vi "Interpolate V-I curve.vi"(3 "Input axes. True: V vs I; False: I vs V":bool=TRUE, 4 "Number of V-sweep periods":dbl=1.0, 5 "Index of desired plot":i32, 6 "Input Multiplot":cluster{dbl[], dbl[]}[](graph)=[{array[601 elements], array[601 elements]}, {[-7e-09, -6.976666666666667e-09, -6.953333333333333e-09, -6.93e-09, -6.906666666666667e-09, -6.883333333333333e-09, -6.86e-09, -6.836666666666667e-09, -6.813333333333333e-09, -6.79e-09, -6.766666666666666e-09, -6.743333333333333e-09, -6.72e-09, -6.696666666666666e-09, -6.673333333333333e-09, -6.65e-09, -6.626666666666666e-09, -6.603333333333333e-09, -6.58e-09, -6.556666666666666e-09, -6.533333333333333e-09, -6.51e-09, -6.486666666666666e-09, -6.463333333333333e-09, -6.44e-09, -6.416666666666666e-09, -6.393333333333333e-09, -6.37e-09, -6.346666666666666e-09, -6.323333333333333e-09, -6.3e-09, -6.276666666666666e-09, -6.253333333333333e-09, -6.23e-09, -6.206666666666666e-09, -6.183333333333333e-09, -6.16e-09, -6.136666666666666e-09, -6.113333333333333e-09, -6.09e-09, -6.066666666666666e-09, -6.043333333333333e-09, -6.02e-09, -5.9966666666666664e-09, -5.973333333333333e-09, -5.9499999999999995e-09, -5.9266666666666665e-09, -5.9033333333333334e-09, -5.8799999999999995e-09, -5.8566666666666665e-09, -5.833333333333333e-09, -5.8099999999999996e-09, -5.7866666666666665e-09, -5.763333333333333e-09, -5.74e-09, -5.7166666666666666e-09, -5.693333333333333e-09, -5.67e-09, -5.646666666666667e-09, -5.623333333333333e-09, -5.6e-09, -5.576666666666667e-09, -5.553333333333333e-09, -5.53e-09, -5.506666666666667e-09, -5.483333333333333e-09, -5.46e-09, -5.436666666666667e-09, -5.413333333333333e-09, -5.39e-09, -5.366666666666667e-09, -5.343333333333333e-09, -5.32e-09, -5.296666666666667e-09, -5.273333333333333e-09], [-0.0004821561460872206, -0.00047938288334669894, -0.0004789074718402786, -0.0004777379416474081, -0.000475052203857136, -0.00047223609393540406, -0.00047195794806430995, -0.0004706001620611257, -0.00046771079567058956, -0.0004666969301809305, -0.00046440072995060437, -0.00046159074960749647, -0.0004603654022456595, -0.00045960525980296877, -0.0004591186437168279, -0.00045718015199764495, -0.00045405957870414866, -0.00045358976275954613, -0.00045141277699479917, -0.00044926701129684773, -0.00044740158603609226, -0.00044689019117776554, -0.00044619043907049053, -0.0004433306418334057, -0.00044036373125306503, -0.0004390323537054179, -0.0004379883109219583, -0.0004348498737591965, -0.0004331149798360703, -0.0004325833412496541, -0.00043100042072116127, -0.0004279667670998173, -0.0004274959945874391, -0.000424231161635493, -0.0004224971179265378, -0.00042197779306206125, -0.00042081665841692983, -0.00041722347727663384, -0.00041579225134809604, -0.0004153896972753539, -0.0004137941384571501, -0.0004143376010798538, -0.00041033705328048575, -0.00040735040411746563, -0.00040853045386952307, -0.0004054030297437131, -0.0004025822771474479, -0.0004006957311862501, -0.0004002209530181583, -0.00039750432495219164, -0.00039564320668351497, -0.0003952796011456548, -0.0003927923532153638, -0.0003905100464353255, -0.0003899183298476656, -0.00038911154346687804, -0.0003854091447564508, -0.0003832058693739394, -0.00038282830855911076, -0.0003796885675621918, -0.00038073464055646787, -0.00037735716246794447, -0.000374384671207582, -0.0003752523277341829, -0.00037167521639979383, -0.0003703811833337198, -0.0003688859978404175, -0.0003683934511922314, -0.0003657335680347226, -0.0003637132236609178, -0.00036318711871480454, -0.00035897924338772544, -0.00035829389578091205, -0.00035748300144421987, -0.0003552158910910105]}, {[-5.599999999999997e-10, -5.366666666666667e-10, -5.133333333333328e-10, -4.899999999999998e-10, -4.666666666666667e-10, -4.4333333333333284e-10, -4.199999999999998e-10, -3.9666666666666674e-10, -3.7333333333333287e-10, -3.499999999999998e-10, -3.266666666666668e-10, -3.033333333333329e-10, -2.7999999999999986e-10, -2.566666666666668e-10, -2.3333333333333294e-10, -2.099999999999999e-10, -1.8666666666666602e-10, -1.6333333333333298e-10, -1.3999999999999993e-10, -1.1666666666666606e-10, -9.333333333333301e-11, -6.999999999999997e-11, -4.666666666666609e-11, -2.3333333333333046e-11, 0.0, 2.3333333333333873e-11, 4.666666666666692e-11, 6.999999999999997e-11, 9.333333333333384e-11, 1.1666666666666688e-10, 1.3999999999999993e-10, 1.633333333333338e-10, 1.8666666666666685e-10, 2.099999999999999e-10, 2.3333333333333377e-10, 2.566666666666668e-10, 2.7999999999999986e-10, 3.0333333333333373e-10, 3.266666666666668e-10, 3.5000000000000065e-10, 3.733333333333337e-10, 3.9666666666666674e-10, 4.200000000000006e-10, 4.4333333333333366e-10, 4.666666666666675e-10, 4.899999999999998e-10, 5.133333333333336e-10, 5.366666666666675e-10, 5.599999999999997e-10, 5.833333333333336e-10], [-1.0908391112264728e-05, -8.644820502116776e-06, -6.8977031689387985e-06, -5.984813208800999e-06, -5.453391200129657e-06, -4.585249992454284e-06, -2.33240487629176e-06, -8.957815403187959e-07, -3.5962628994854835e-07, -6.075505381543924e-08, 1.8604182865815456e-06, 2.841798426668403e-06, 4.249988829266792e-06, 4.715480765009576e-06, 6.227967413831692e-06, 7.668111990986195e-06, 8.239208285420787e-06, 8.970385450334904e-06, 1.0901477984742562e-05, 1.1938842152533559e-05, 1.2519419028859791e-05, 1.3099995905186172e-05, 1.3977921007139181e-05, 1.6099870634156064e-05, 1.7178893430687366e-05, 1.7754762256515482e-05, 1.8375476226263603e-05, 1.955084525086182e-05, 2.1566626045237013e-05, 2.2327165677538652e-05, 2.2693563802318587e-05, 2.3746583450759822e-05, 2.653313810987007e-05, 2.6961992026978492e-05, 2.739084594408704e-05, 2.912436894680552e-05, 3.0129040728652255e-05, 2.9961392877854862e-05, 3.24601919222609e-05, 3.3679911675141054e-05, 3.571628210662536e-05, 3.6257532921809454e-05, 3.704406684689527e-05, 3.88762069054447e-05, 4.038245121009152e-05, 4.0933599608131805e-05, 4.1661639815733367e-05, 4.3197892351489786e-05, 4.543482864557507e-05, 4.602267755767849e-05]}]) -> (0 "dt (dxi) output":dbl=2.325555555555556e-11, 1 "Suggested SC Offset":dbl, 2 "Interpolated Plot":cluster{"xi used":dbl[], "yi":dbl[]}(graph))   [LabVIEW 2016]
uses:
  <vilib>/gmath/NI_Gmath.lvlib
  <vilib>/Analysis/NI_AALPro.lvlib
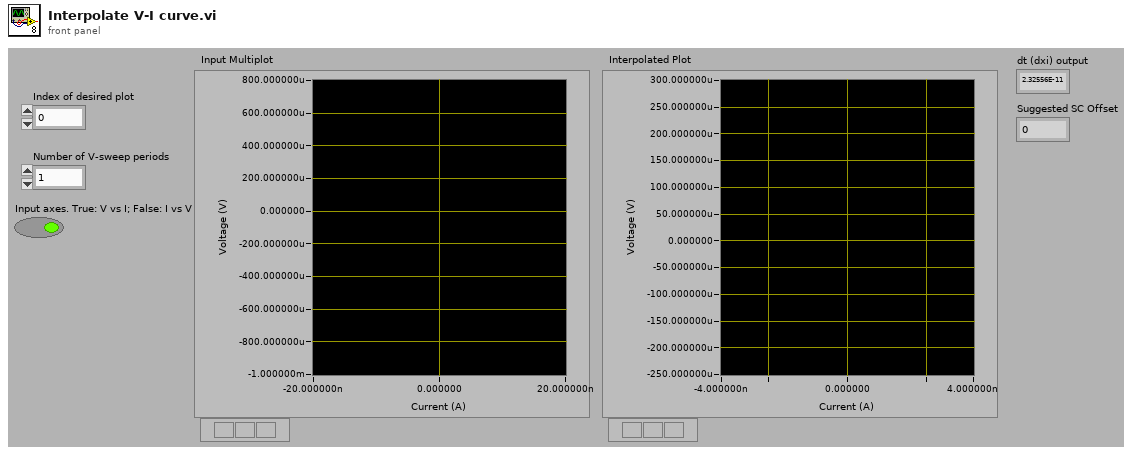
[diagram p1: front panel]
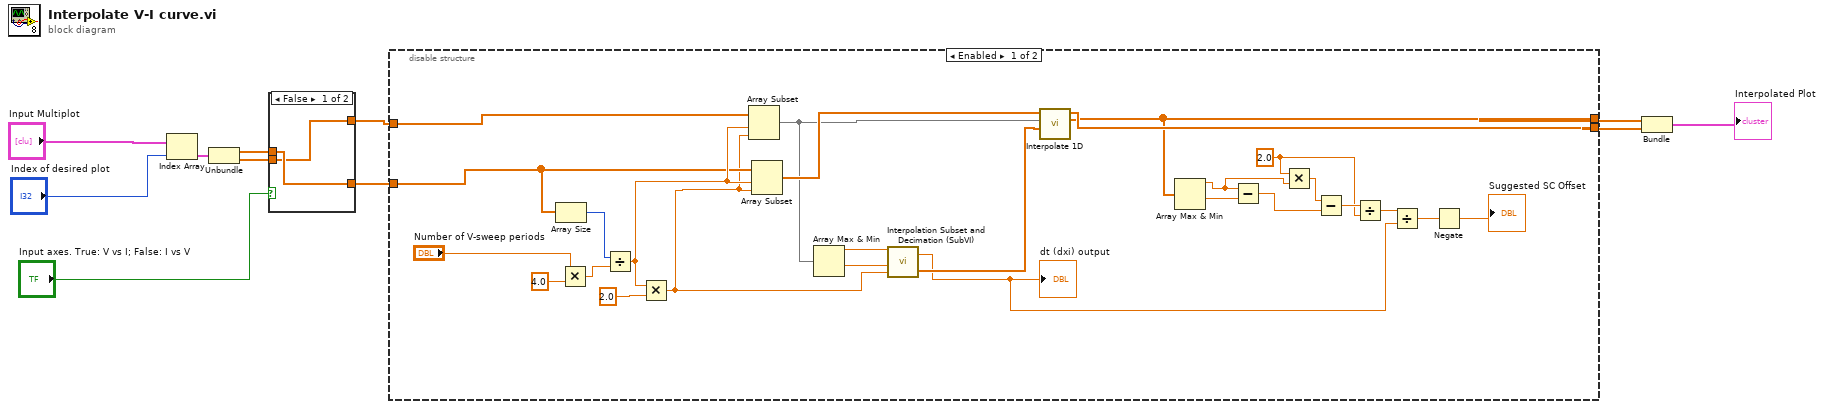
[diagram p0: block diagram]
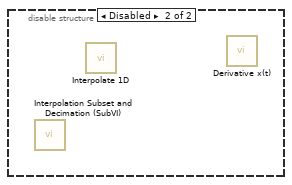
[diagram p3: hidden frame]
diagram:
  n1 = Index Array(array="Input Multiplot", index="Index of desired plot") -> (element=w10:cluster{dbl[], dbl[]})
  n2 = Unbundle(w10) -> (w4:dbl[], w3:dbl[])
  n3 = case shown="False" "Input axes. True: V vs I; False: I vs V" {
    tunnel: [w12 w15] -> w5
    tunnel: w4 -> [w13 w15]
    tunnel: w3 -> [w12 w14]
    tunnel: [w13 w14] -> w2
    frame False {
    }
    frame True {
    }
  }
  n4 = disable-structure shown="Enabled" {
    disable-tunnel: w5 -> [w35 _]
    disable-tunnel: w2 -> [w34 _]
    disable-tunnel: [w31 _] -> w9
    disable-tunnel: [w26 _] -> w8
    frame Enabled {
      w20 = 2.0 ("x")
      n5 = Array Size(array=w34) -> (size(s)=w36:i32)
      n6 = Multiply(x="Number of V-sweep periods", y=4.0) -> (x*y=w38:dbl)
      n7 = Divide(x=w36, y=w38) -> (x/y=w37:dbl)
      n8 = Multiply(x=w37, y=2.0) -> (x*y=w27:dbl)
      n9 = Array Subset(array=w35, index=w37, length=w27) -> (w30:dbl[])
      n10 = Array Subset(array=w34, index=w37, length=w27) -> (w33:dbl[])
      n11 = Array Max & Min(array=w30) -> (max value=w29:dbl, min value=w28:dbl)  [unwired: 2 out]
      n12 = call "Interpolation Subset and Decimation (SubVI).vi"("decimation points"=w27, "Low value"=w28, "High value"=w29) -> ("Points to use in interpolation (xi)"=w32:dbl[], "Numeric"=w18:dbl)
      "dt (dxi) output" <- w18
      n13 = call <vilib>:"Interpolate 1D.vi"("xi"=w32, "X"=w30, "Y"=w33) -> ("xi used"=w26:dbl[], "yi"=w31:dbl[])  [unwired: 6 in, 1 out]
      n14 = Array Max & Min(array=w26) -> (max value=w24:dbl, min value=w25:dbl)  [unwired: 2 out]
      n15 = Subtract(x=w24, y=w25) -> (x-y=w22:dbl)
      n16 = Multiply(x=w20, y=w24) -> (x*y=w23:dbl)
      n17 = Subtract(x=w23, y=w22) -> (x-y=w21:dbl)
      n18 = Divide(x=w21, y=w20) -> (x/y=w19:dbl)
      n19 = Divide(x=w19, y=w18) -> (x/y=w17:dbl)
      n20 = Negate(x=w17) -> (-x=→"Suggested SC Offset":dbl)
    }
    frame Disabled {
      n21 = call "Interpolation Subset and Decimation (SubVI).vi"() -> ()  [unwired: 3 in, 2 out]
      n22 = call <vilib>:"Interpolate 1D.vi"() -> ()  [unwired: 9 in, 3 out]
      n23 = call <vilib>:"Derivative x(t).vi"() -> ()  [unwired: 10 in, 2 out]
    }
  }
  n24 = Bundle("xi used"=w8, "yi"=w9) -> (→"Interpolated Plot":cluster{"xi used":dbl[], "yi":dbl[]})  [unwired: 1 in]
